vi "Level Color.vi"(10 "Numeric Indicator Reference":refnum<vi>, 11 "LVL Chart Refernce":refnum<vi>) -> ()   [LabVIEW 2016, in "Instrument.OxfordVRM UI.lvclass"]
uses:
  Instrument.OxfordVRM UI.lvclass
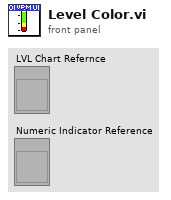
[diagram p1: front panel]
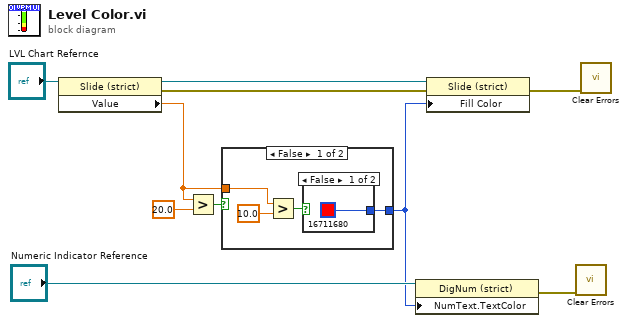
[diagram p0: block diagram]
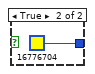
[diagram p2: hidden frame]
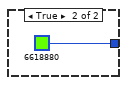
[diagram p3: hidden frame]
diagram:
  n1 = property on="Property Node" class="Slide (strict)"(reference="LVL Chart Refernce") -> (reference out=w9:refnum<vi>, error out=w4:errorcluster, "Value"=w1:dbl)  [unwired: 1 in]
  n2 = Greater?(x=w1, y=20.0) -> (0:w5:bool)
  n3 = case shown="False" w5 {
    tunnel: [w14 u32 6618880] -> w7
    tunnel: w1 -> [w11 _]
    frame False {
      n4 = Greater?(x=w11, y=10.0) -> (0:w12:bool)
      n5 = case shown="False" w12 {
        tunnel: [u32 16711680 u32 16776704] -> w14
        frame False {
        }
        frame True {
        }
      }
    }
    frame True {
    }
  }
  n6 = property on="Property Node" class="DigNum (strict)"(reference="Numeric Indicator Reference", "NumText.TextColor"=w7) -> (error out=w2:errorcluster)  [unwired: 1 in, 1 out]
  n7 = property on="Property Node" class="Slide (strict)"(reference=w9, error in=w4, "Fill Color"=w7) -> (error out=w3:errorcluster)  [unwired: 1 out]
  n8 = call <vilib>:"Clear Errors.vi"("error in (no error)"=w2) -> ()  [unwired: 5 in, 2 out]
  n9 = call <vilib>:"Clear Errors.vi"("error in (no error)"=w3) -> ()  [unwired: 5 in, 2 out]
